vi "Refresh Configuration.vi"(8 "error in":errorcluster, 11 "Config in":refnum<class "Config.lvclass">) -> (0 "error out":errorcluster, 3 "Config out":refnum<class "Config.lvclass">)   [LabVIEW 2023, in "Config.lvlib" / "Config.lvclass"]
uses:
  Config.lvclass
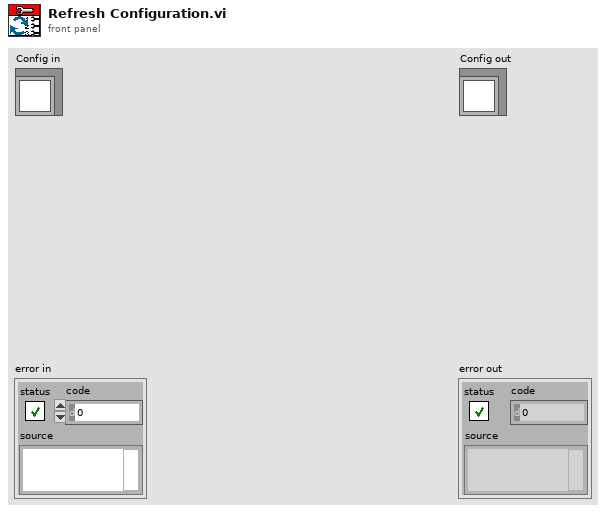
[diagram p1: front panel]
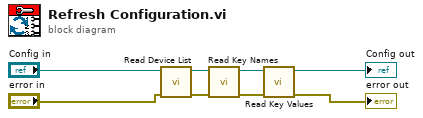
[diagram p0: block diagram]
diagram:
  n1 = call "Read Device List.vi"("error in"="error in", "Config in"="Config in") -> ("error out"=w7:errorcluster, "Config out"=w5:refnum<class "Config.lvclass">)  [unwired: 7 in, 1 out]
  n2 = call "Read Key Names.vi"("error in"=w7, "Config in"=w5) -> ("error out"=w8:errorcluster, "Config out"=w6:refnum<class "Config.lvclass">)  [unwired: 8 in]
  n3 = call "Read Key Values.vi"("error in"=w8, "Config in"=w6) -> ("error out"=→"error out":errorcluster, "Config out"=→"Config out":refnum<class "Config.lvclass">)  [unwired: 8 in]
